vi "iV programa 2_1.vi"() -> ()   [LabVIEW 2020]
panel:
  out "Array":dbl[](array[numeric])
  out "Element no:":dbl
  in  "Ingrese el numero de elementos \nde la secuencia":i8
  out "Fibonacci secuence":i32
  # "2.1. Elabore un código que muestre en un arreglo la serie numérica de Fibonacci. Considere lo siguiente:\n• Un control de le permita al usuario determinar la cantidad de elementos a guardar en el arreglo.\n• Un indicador para la serie. Si elige mostrar la serie en un indicador escalar, \ndeberá agregar el tiempo necesaria para poder visualizar el cambio."
  # "Secuencia fibonacci: 1, 1, 2, 3, 5, 8, 13, 21, 34, 55, 89, 144, 233, 377..."
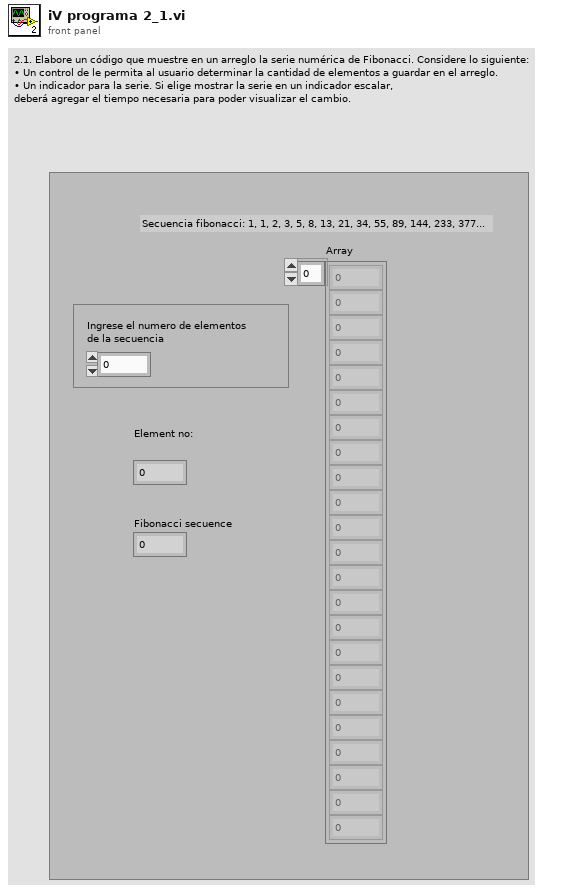
[diagram p1: front panel]
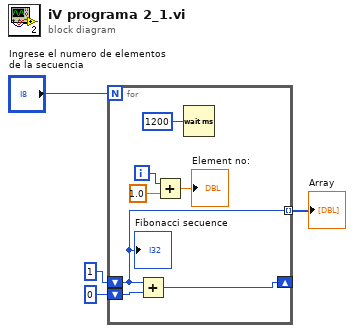
[diagram p0: block diagram]
diagram:
  n1 = for {
    N: "Ingrese el numero de elementos \nde la secuencia" -> [_]
    shift-right: [w10] -> _
    shift-left: 1 -> [w5]
    shift-left: 0 -> [w11]
    tunnel: [w5] -> w1 mode=indexing
    i -> [w7]
    n2 = Add(x=w5, y=w11) -> (x+y=w10:i32)
    n3 = Add(x=w7, y=1.0) -> (x+y=→"Element no:":dbl)
    n4 = Wait (ms)(milliseconds to wait=u32 1200) -> ()  [unwired: 1 out]
    "Fibonacci secuence" <- w5
  }
  "Array" <- w1
